vi "list cameras.vi"(8 "error in (no error)":errorcluster) -> (0 "error out":errorcluster, 2 "Cameras":T1[](array[typedef]))   [LabVIEW 2022 SP3, in "Vision.lvlib"]
uses:
  Vision.lvlib
  camera.ctl
  camera driver.ctl
  C:/Users/Caleb/Desktop/nebraska-silicon-lab/pixel-gantry-extra/LV/bin/uEyeDotNet.dll
  bin/uEyeDotNet.dll
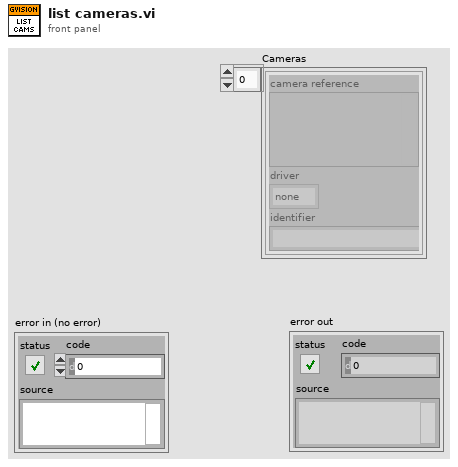
[diagram p1: front panel]
types:
  T1 = typedef "Vision.lvlib/camera.ctl" = cluster{"camera reference":variant, "driver":T2, "identifier":string}
  T2 = typedef "Vision.lvlib/camera driver.ctl" = enum16{"none", "ueye", "escapi"}
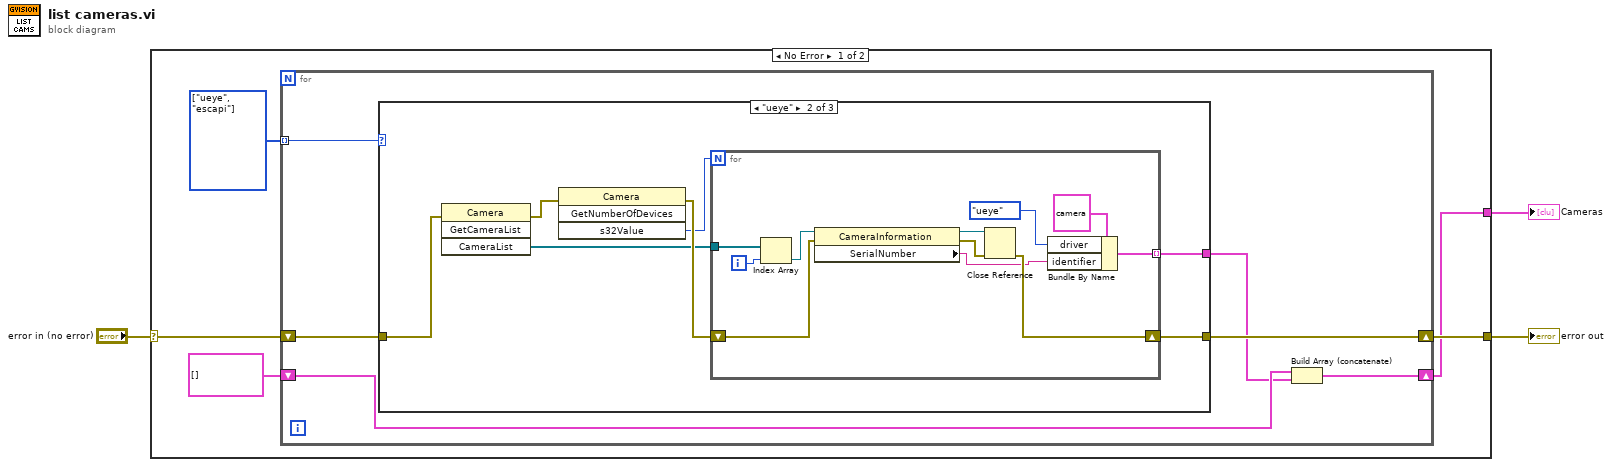
[diagram p0: block diagram]
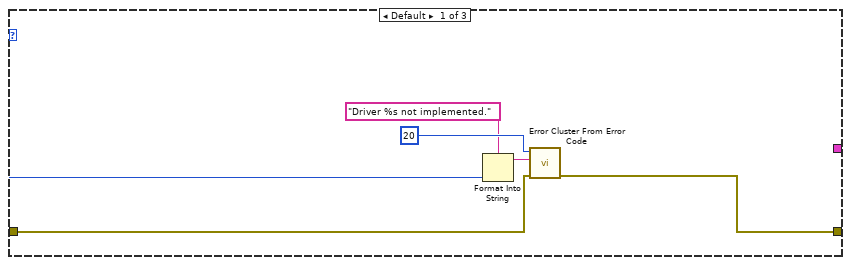
[diagram p2: hidden frame]
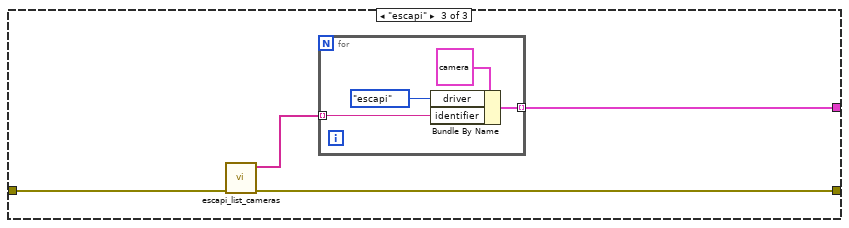
[diagram p3: hidden frame]
diagram:
  n1 = case shown="No Error" "error in (no error)" {
    selector: "error in (no error)" -> [w8 w47]
    tunnel: [w7 w47] -> w2
    tunnel: [w4 _] -> w1
    frame No Error {
      w6 = T2[] [enum."ueye", enum."escapi"] items=["none", "ueye", "escapi"]
      n2 = for {
        shift-right: [w13] -> w7
        shift-left: w8 -> [w14]
        tunnel: w6 -> [w12] mode=indexing
        shift-right: [w9] -> w4
        shift-left: T1[] [] -> [w11]
        n3 = case shown="\"ueye\"" w12 {
          selector: w12 -> [w16 _ _]
          tunnel: w14 -> [w19 w27 w42]
          tunnel: [w18 w24 w39] -> w13
          tunnel: [_ w21 w40] -> w10
          frame Default {
            n4 = Format Into String(format string="Driver %s not implemented.", w16) -> (resulting string=w15:string)  [unwired: 2 in, 1 out]
            n5 = call <vilib>:"Error Cluster From Error Code.vi"("error in (no error)"=w19, "error message (\"\")"=w15, "error code (0)"=20) -> ("error out"=w18:errorcluster)  [unwired: 6 in]
          }
          frame "ueye" {
            n6 = invoke on="Methodenknoten" class="Camera" method="GetCameraList"(error in=w27) -> (error out=w26:errorcluster, "CameraList"=w23:refnum<k24>[])  [unwired: 3 in, 2 out]
            n7 = invoke on="Methodenknoten" class="Camera" method="GetNumberOfDevices"(error in=w26) -> (error out=w25:errorcluster, "s32Value"=w22:i32)  [unwired: 3 in, 2 out]
            n8 = for {
              N: w22 -> [_]
              shift-right: [w32] -> w24
              shift-left: w25 -> [w34]
              tunnel: w23 -> [w38]
              tunnel: [w28] -> w21 mode=indexing
              i -> [w37]
              n9 = Index Array(array=w38, index=w37) -> (element=w35:refnum<k24>)
              n10 = property class="CameraInformation"(reference=w35, error in=w34) -> (reference out=w36:refnum<k24>, error out=w33:errorcluster, "SerialNumber"=w31:string)
              n11 = Close Reference(reference=w36, error in (no error)=w33) -> (error out=w32:errorcluster)
              n12 = Bundle By Name(cluster=T1 {"camera reference"=variant, "driver"=enum."none", "identifier"=""}, "driver"=camera_driver."ueye", "identifier"=w31) -> (w28:T1)
            }
          }
          frame "escapi" {
            n13 = call "escapi_list_cameras.vi"("error in (no error)"=w42) -> ("error out"=w39:errorcluster, "Cam Names"=w41:string[])  [unwired: 9 in]
            n14 = for {
              tunnel: w41 -> [w44] mode=indexing
              tunnel: [w43] -> w40 mode=indexing
              n15 = Bundle By Name(cluster=T1 {"camera reference"=variant, "driver"=enum."none", "identifier"=""}, "driver"=camera_driver."escapi", "identifier"=w44) -> (w43:T1)
            }
          }
        }
        n16 = Build Array (concatenate)(w11, w10) -> (w9:T1[])
      }
    }
    frame Error {
    }
  }
  "error out" <- w2
  "Cameras" <- w1
